vi "Drivetrain Loop.vi"() -> ()   [LabVIEW 2015]
uses:
  Common Code/Drivetrain Modes.ctl
  Robot Global Data.vi
  <vilib>/Rock Robotics/WPI/Solenoid/Deprecated/WPI_SolenoidSetBool.vi
  <vilib>/Rock Robotics/Network Tables/NT Write Number.vi
panel:
  out "Modes":T1=enum."Vision Targeting"
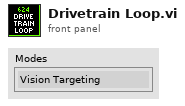
[diagram p1: front panel]
types:
  T1 = typedef "Drivetrain Modes.ctl" = enum16{"Climb", "Manual", "Vision Targeting", "PID Distance Drive", "Hybrid"}
  T2 = typedef "Drivetrain Commands.ctl" = cluster{"Y Power":dbl, "Turn Power":dbl, "Distance":dbl, "Manual AQ?":bool, "1st Gear?":bool, "Modes":T1}
  T3 = typedef "WPI_SolenoidDevRef.ctl" = cluster{"DevStatus":errorcluster, "Pneumatics Control Module":u8, "Forward Solenoid Channel":T4, "Reverse Solenoid Channel":T4}
  T4 = typedef "WPI_SolenoidChannel.ctl" = enum8{"Solenoid 0", "Solenoid 1", "Solenoid 2", "Solenoid 3", "Solenoid 4", "Solenoid 5", "Solenoid 6", "Solenoid 7", "Invalid"}
  T5 = typedef "Drivetrain Status Cluster.ctl" = cluster{"Modes":T1, "Y (Throttle)":dbl, "X (Steer)":dbl}
  T6 = typedef "WPI_MotorControlDeviceRef.ctl" = cluster{"DeviceStatus":errorcluster, "Type":T7, "PWM":cluster{"PWM Channel":T8, "DeadBand":T9}, "CAN":cluster{"Device Number":u8, "Control Mode":T10, "Semaphore":T11, "Max Vout":dbl, "TalonSRX Control Mode":T12}, "Invert":bool}
  T7 = typedef "WPI_MotorControlType.ctl" = enum16{"PWM", "CAN", "CANTalonSRX"}
  T8 = typedef "FPGA_DIOPWMChannel.ctl" = enum8{"PWM 0", "PWM 1", "PWM 2", "PWM 3", "PWM 4", "PWM 5", "PWM 6", "PWM 7", "PWM 8", "PWM 9", "PWM MXP 0", "PWM MXP 1", "PWM MXP 2", "PWM MXP 3", "PWM MXP 4", "PWM MXP 5", "PWM MXP 6", "PWM MXP 7", "PWM MXP 8", "PWM MXP 9", "Invalid"}
  T9 = typedef "WPI_PWMDeadband.ctl" = cluster{"Name":string, "maxPositivePwm":i32, "minPositivePwm":i32, "centerPwm":i32, "maxNegativePwm":i32, "minNegativePwm":i32, "angularRange":u16}
  T10 = typedef "WPI_CANJaguar_ControlMode.ctl" = enum8{"Percent VBus", "Current", "Speed", "Position", "Voltage"}
  T11 = typedef "Semaphore RefNum" = refnum<k1>
  T12 = typedef "WPI_CANTalonSRX_APIControlMode.ctl" = enum8{"Percent VBus", "Speed", "Position", "Slave", "Unchanged / Invalid", "Voltage Compensation", "Current", "Motion Profile"}
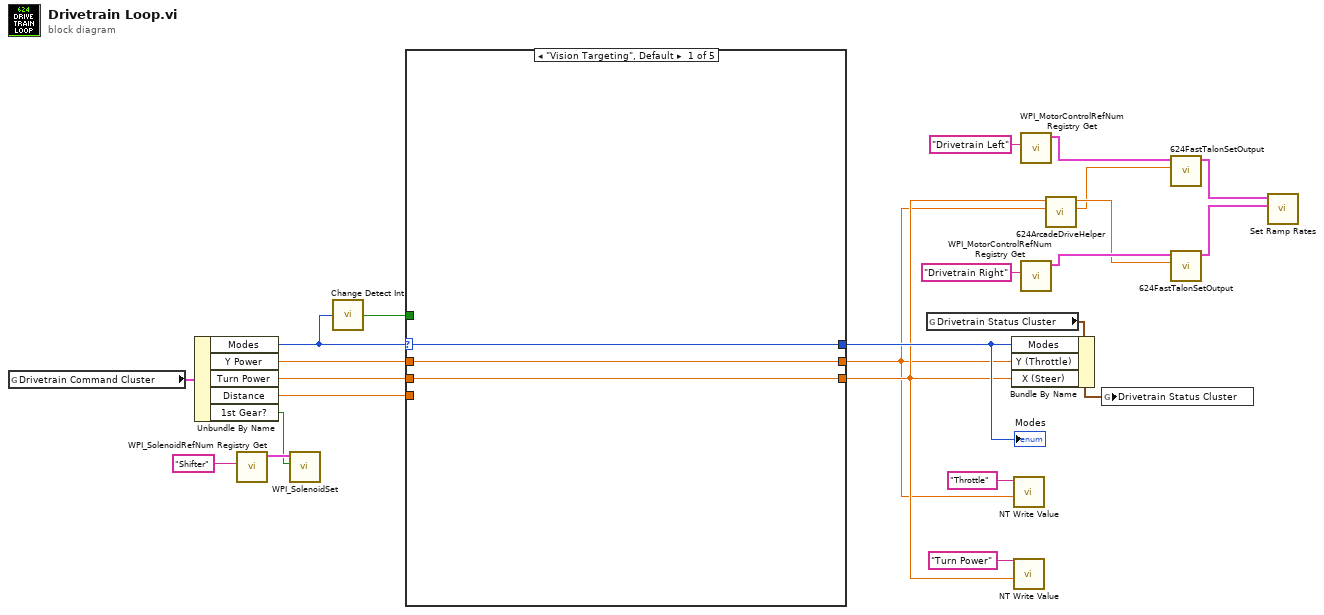
[diagram p0: block diagram]
diagram:
  n1 = global read "Robot Global Data.vi" "Drivetrain Command Cluster"() -> (w24:T2)
  n2 = Unbundle By Name(w24) -> ("Modes"=w11:T1, "Y Power"=w23:dbl, "Turn Power"=w22:dbl, "Distance"=w21:dbl, "1st Gear?"=w18:bool)
  n3 = call <vilib>:"WPI_SolenoidRefNum Registry Get.vi"("refnum name"="Shifter") -> ("SolenoidDevRef"=w19:T3)  [unwired: 9 in, 1 out]
  n4 = call-poly <vilib>:"WPI_SolenoidSet.vi"("Value"=w18, "SolenoidDevRef"=w19) -> ()  [unwired: 8 in, 2 out]
  n5 = call "Change Detect Int.vi"("In"=w11) -> ("Changed?"=w10:bool)
  n6 = case shown="\"Vision Targeting\", Default" w11 {
    selector: w11 -> [w27 w28 _ w31 _]
    tunnel: w23 -> [w26 _ _ w30 _]
    tunnel: w22 -> [w25 _ _ w29 _]
    tunnel: w21 -> [_ _ _ _ _]
    tunnel: [w26 _ _ w30 _] -> w3
    tunnel: [w25 _ _ w29 _] -> w4
    tunnel: [w27 w28 _ w31 _] -> w15
    tunnel: w10 -> [_ _ _ _ _]
    frame "Vision Targeting", Default {
    }
    frame "PID Distance Drive" {
    }
    frame "Hybrid" {
    }
    frame "Manual" {
    }
    frame "Climb" {
    }
  }
  "Modes" <- w15
  n7 = global read "Robot Global Data.vi" "Drivetrain Status Cluster"() -> (w17:T5)
  n8 = Bundle By Name(cluster=w17, "Modes"=w15, "Y (Throttle)"=w3, "X (Steer)"=w4) -> (w16:T5)
  n9 = call-poly <vilib>:"NT Write Value.vi"("Numeric"=w3, "Name"="Throttle") -> ()  [unwired: 9 in, 1 out]
  n10 = call-poly <vilib>:"NT Write Value.vi"("Numeric"=w4, "Name"="Turn Power") -> ()  [unwired: 9 in, 1 out]
  n11 = call <vilib>:"WPI_MotorControlRefNum Registry Get.vi"("refnum name"="Drivetrain Left") -> ("MotorControlDevRef"=w8:T6)  [unwired: 9 in, 1 out]
  n12 = call <vilib>:"WPI_MotorControlRefNum Registry Get.vi"("refnum name"="Drivetrain Right") -> ("MotorControlDevRef"=w9:T6)  [unwired: 9 in, 1 out]
  n13 = call "624ArcadeDriveHelper.vi"("Y Power"=w3, "Turn Power"=w4) -> ("Left"=w1:dbl, "Right"=w2:dbl)  [unwired: 8 in]
  n14 = global write "Robot Global Data.vi" "Drivetrain Status Cluster"(w16) -> ()
  n15 = call "624FastTalonSetOutput.vi"("Output"=w1, "MotorControlDevRef"=w8) -> ("MotorControlDevRef"=w7:T6)  [unwired: 8 in, 1 out]
  n16 = call "624FastTalonSetOutput.vi"("Output"=w2, "MotorControlDevRef"=w9) -> ("MotorControlDevRef"=w6:T6)  [unwired: 8 in, 1 out]
  n17 = call "Set Ramp Rates.vi"("DT Right"=w6, "DT Left"=w7) -> ()  [unwired: 10 in]
